vi "daqio_Get_All_Channel_Types.vi"(8 "error in (no error)":errorcluster, 11 "daq.io type in":T2={"daq.io ref"=refnum, "daq.io API Base"="http://dashboard.daq.io/api/v1", "Device Type Key"="", "Device Key"="", "Account ID"="", "online"=TRUE}) -> (0 "error out":errorcluster, 2 "All Channel Types":T1[](array[typedef]), 3 "daq.io type out":T2={"daq.io ref"=refnum, "daq.io API Base"="http://dashboard.daq.io/api/v1", "Device Type Key"="", "Device Key"="", "Account ID"="", "online"=TRUE})   [LabVIEW 2013, in "daqio minimal.lvlib"]
doc: "This VI returns all Channel Types for a specific Device Type."
uses:
  daqio minimal.lvlib
  _typedefs/daqio-Type.ctl
  <vilib>/httpClient/ClientHandle.ctl
  _typedefs/daqio-Channel-Type-POST-return.ctl
  <vilib>/Easy HTTP Client/Easy HTTP.lvlib
  <vilib>/httpClient/LabVIEWHTTPClient.lvlib
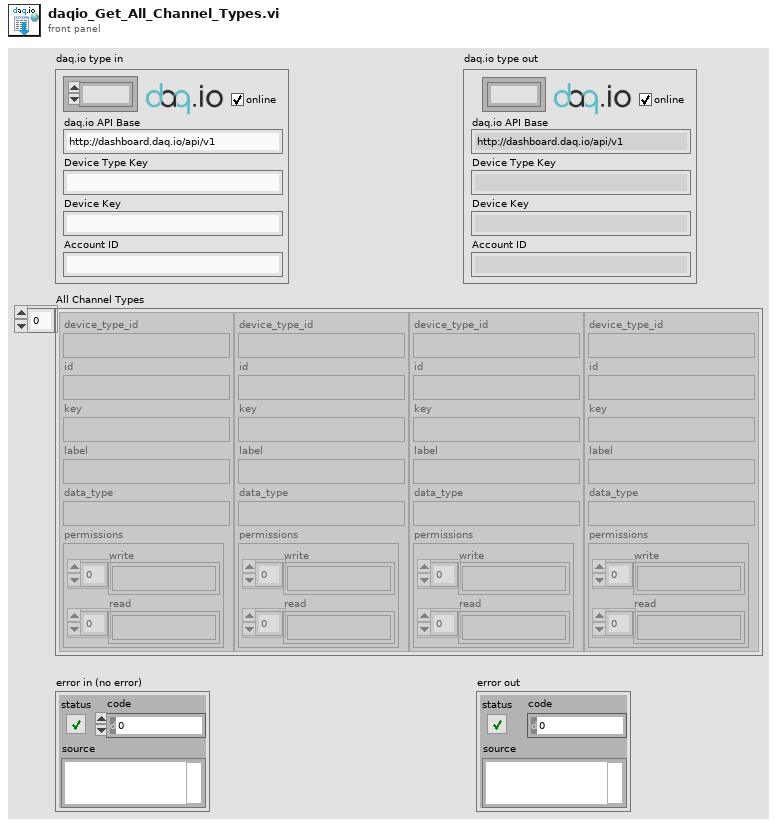
[diagram p1: front panel]
types:
  T1 = typedef "daqio minimal.lvlib/daqio-Channel-Type-POST-return.ctl" = cluster{"device_type_id":string, "id":string, "key":string, "label":string, "data_type":string, "permissions":cluster{"write":string[], "read":string[]}}
  T2 = typedef "daqio minimal.lvlib/daqio-Type.ctl" = cluster{"daq.io ref":T3, "daq.io API Base":string, "Device Type Key":string, "Device Key":string, "Account ID":string, "online":bool}
  T3 = typedef "LabVIEWHTTPClient.lvlib/ClientHandle.ctl" = refnum<k1>
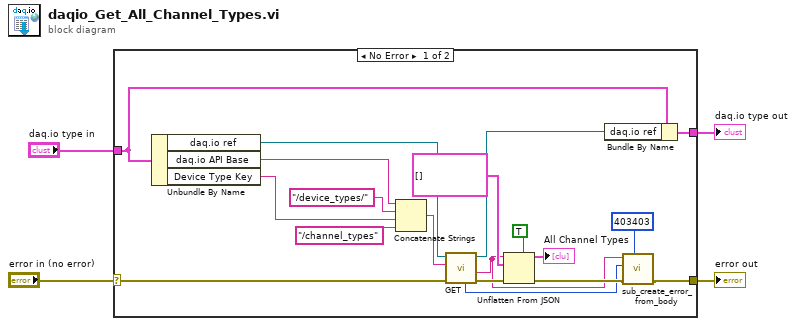
[diagram p0: block diagram]
diagram:
  n1 = case shown="No Error" "error in (no error)" {
    selector: "error in (no error)" -> [w16 w24]
    tunnel: "daq.io type in" -> [w21 w25]
    tunnel: [w20 w25] -> w3
    tunnel: [w9 w24] -> w2
    frame No Error {
      n2 = Unbundle By Name(w21) -> ("daq.io ref"=w18:T3, "daq.io API Base"=w19:string, "Device Type Key"=w14:string)
      n3 = Concatenate Strings(w19, "/device_types/", w14, "/channel_types") -> (w13:string)
      n4 = call <vilib>:"GET.vi"("error in (no error)"=w16, "url"=w13, "client handle"=w18) -> ("error out"=w15:errorcluster, "body"=w6:string, "client handle out"=w17:T3, "HTTP Response Code"=w7:i32)  [unwired: 4 in, 1 out]
      n5 = Unflatten From JSON(enable LabVIEW extensions? (T)=TRUE, JSON string=w6, type and defaults=T1[] [], error in (no error)=w15) -> (value=→"All Channel Types":T1[], error out=w10:errorcluster)  [unwired: 3 in]
      n6 = Bundle By Name(cluster=w21, "daq.io ref"=w17) -> (w20:T2)
      n7 = call "sub_create_error_from_body.vi"("error code"=403403, "error in (no error)"=w10, "http code"=w7, "body"=w6) -> ("error out"=w9:errorcluster)  [unwired: 7 in]
    }
    frame Error {
    }
  }
  "error out" <- w2
  "daq.io type out" <- w3
